vi "MatrixConfiguration.vi"() -> ()   [LabVIEW 2013]
uses:
  InstrControl/InstrumentSetup.vi
  InstrControl/InstrControl.lvclass
panel:
  in  "OK Button":bool
  in  "Apply":bool
  in  "No Matrix":bool
  in  "Save Settings":bool
  in  "Measurement":T1(ring)
  in  "Tab Control":enum32{"Pickering Matrix"}(tab)
  out "Y Mapping":string[](array[string])
  out "X Mapping":string[](array[string])
  out "Display Pickering Matrix":bool[][](array[boolean])
  out "DIAGNOSTIC? Response":string
  in  "Pickering DIAGNOSTIC?":bool
  in  "Pickering Mux2 address":i32=5 caption="Mux2 address"
  in  "Pickering Mux1 address":i32=4 caption="Mux1 address"
  in  "Pickering GPIB address":string caption="GPIB address"
  in  "Pickering Matrix address":i32=1 caption="Matrix address"
  out "X Mapping CB Standard":string[](array[string])
  # "MUX / Matrix Setup"
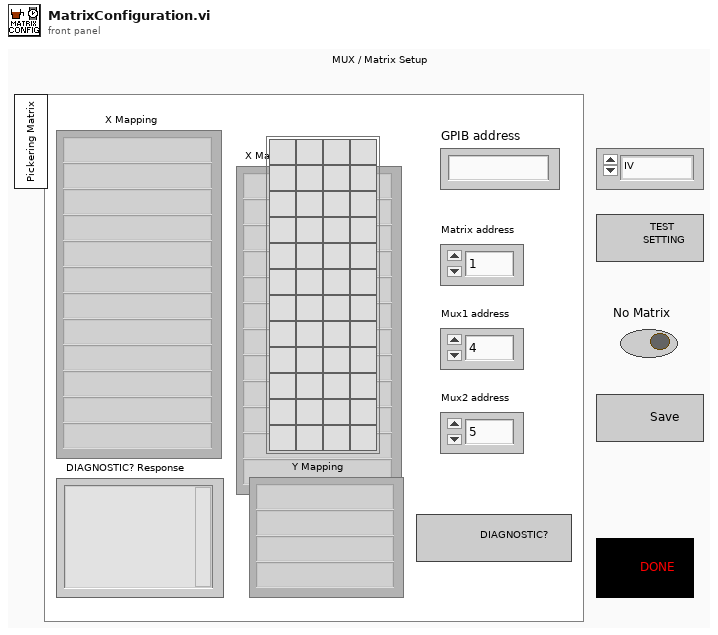
[diagram p1: front panel]
types:
  T1 = enum16{"IV", "CV", "Stability", "Striptest", "Cis", "Ris", "PTP"}
  T2 = enum16{"Reset", "Ground", "Striptest SMU", "Striptest LCR", "IV", "CV", "Interstrip Cap", "Interstrip Res"}
  T3 = cluster{"Matrix address":string, "Mux1 address":string, "Mux2 address":string, "Matrix used?":bool, "Pickering":refnum<class "Pickering.lvclass">, "Matrix X Channels":cluster{"Bias Supply / SMU LO":i32, "Bias Supply / SMU HI":i32, "CV Box LO":i32, "CV Box HI":i32, "CV Box LO IN":i32, "CV Box HI IN":i32, "Volt meter LO":i32, "Volt meter HI":i32, "Mux1 C1":i32, "Mux1 C2":i32, "Mux2 C1":i32, "Mux2 C2":i32}}
  T4 = enum16{"Left Button", "Center Button", "Right Button", "Window Close"}
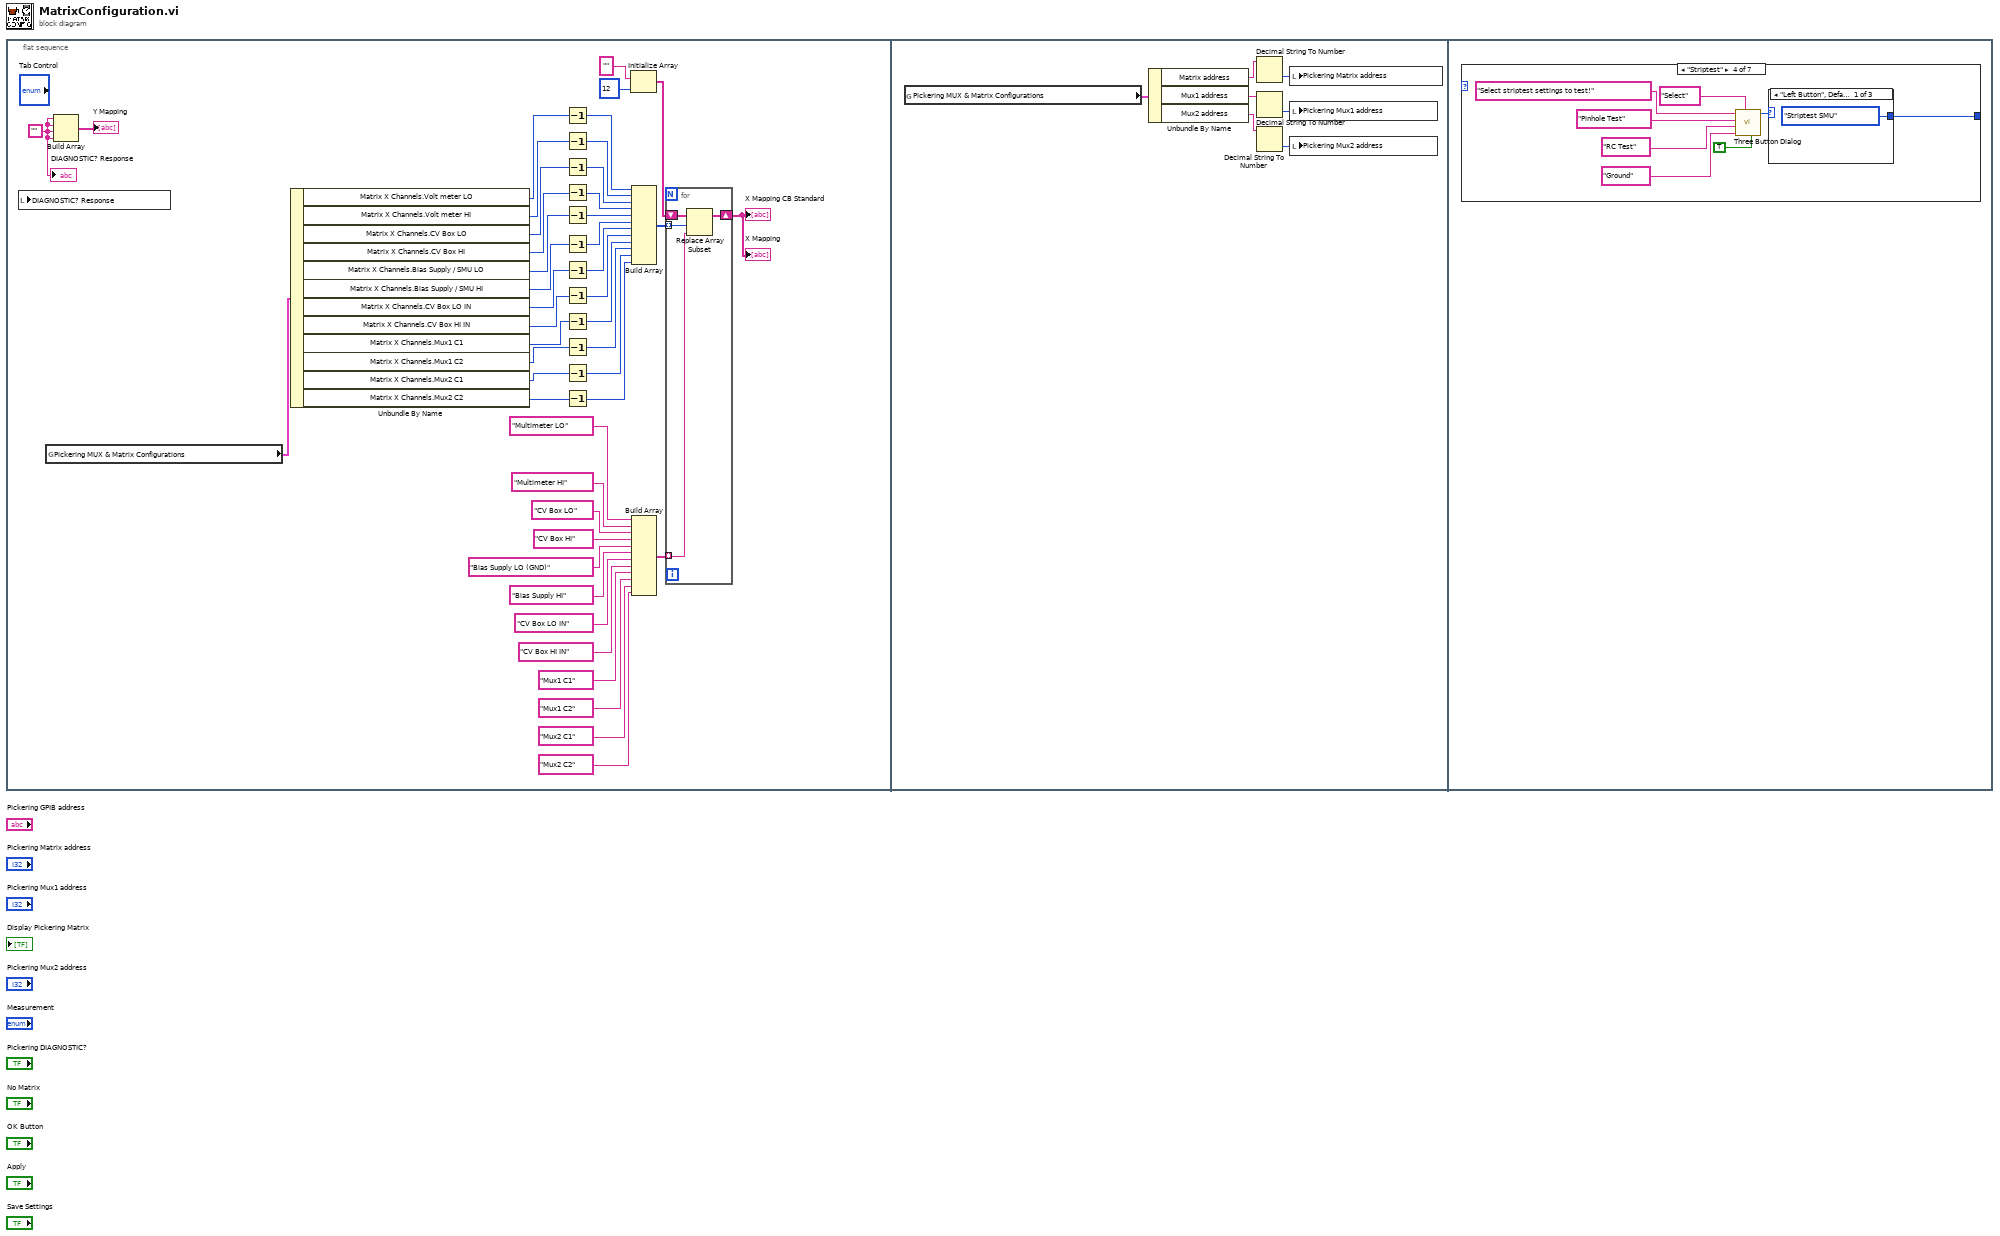
[diagram p0: block diagram]
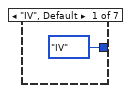
[diagram p2: hidden frame]
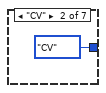
[diagram p3: hidden frame]
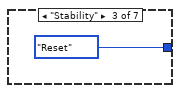
[diagram p4: hidden frame]
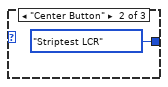
[diagram p5: hidden frame]
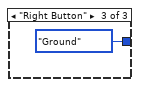
[diagram p6: hidden frame]
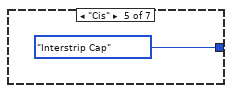
[diagram p7: hidden frame]
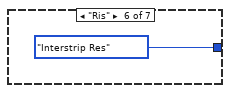
[diagram p8: hidden frame]
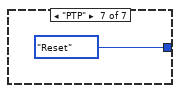
[diagram p9: hidden frame]
diagram:
  n1 = flat-sequence {
    frame #0 {
      w1 = ""
      n2 = local read "DIAGNOSTIC? Response"() -> ()  [unwired: 1 in]
      n3 = global read "InstrumentSetup.vi" "Pickering MUX & Matrix Configurations"() -> (w17:T3)
      n4 = Build Array(w1, w1, w1, w1) -> (→"Y Mapping":string[])
      n5 = Unbundle By Name(w17) -> ("Matrix X Channels.Volt meter LO"=w27:i32, "Matrix X Channels.Volt meter HI"=w29:i32, "Matrix X Channels.CV Box LO"=w18:i32, "Matrix X Channels.CV Box HI"=w23:i32, "Matrix X Channels.Bias Supply / SMU LO"=w22:i32, "Matrix X Channels.Bias Supply / SMU HI"=w21:i32, "Matrix X Channels.CV Box LO IN"=w20:i32, "Matrix X Channels.CV Box HI IN"=w19:i32, "Matrix X Channels.Mux1 C1"=w26:i32, "Matrix X Channels.Mux1 C2"=w25:i32, "Matrix X Channels.Mux2 C1"=w24:i32, "Matrix X Channels.Mux2 C2"=w4:i32)
      n6 = Decrement(x=w27) -> (x-1=w28:i32)
      n7 = Decrement(x=w29) -> (x-1=w30:i32)
      n8 = Decrement(x=w18) -> (x-1=w31:i32)
      n9 = Decrement(x=w23) -> (x-1=w32:i32)
      n10 = Decrement(x=w22) -> (x-1=w33:i32)
      n11 = Decrement(x=w21) -> (x-1=w34:i32)
      n12 = Decrement(x=w20) -> (x-1=w35:i32)
      n13 = Decrement(x=w19) -> (x-1=w36:i32)
      n14 = Decrement(x=w26) -> (x-1=w37:i32)
      n15 = Decrement(x=w25) -> (x-1=w38:i32)
      n16 = Decrement(x=w24) -> (x-1=w39:i32)
      n17 = Decrement(x=w4) -> (x-1=w40:i32)
      n18 = Initialize Array("", 12) -> (w45:string[])
      n19 = Build Array(w28, w30, w31, w32, w33, w34, w35, w36, w37, w38, w39, w40) -> (w41:i32[])
      n20 = Build Array("Multimeter LO" ("Input Element"), "Multimeter HI" ("Input Element"), "CV Box LO" ("Input Element"), "CV Box HI" ("Input Element"), "Bias Supply LO (GND)" ("Input Element"), "Bias Supply HI" ("Input Element"), "CV Box LO IN" ("Input Element"), "CV Box HI IN" ("Input Element"), "Mux1 C1" ("String"), "Mux1 C2" ("String"), "Mux2 C1" ("String"), "Mux2 C2" ("String")) -> (w42:string[])
      n21 = for {
        tunnel: w41 -> [w47] mode=indexing
        tunnel: w42 -> [w48] mode=indexing
        shift-right: [w46] -> w3
        shift-left: w45 -> [w49]
        n22 = Replace Array Subset(array=w49, new element=w48, index=w47) -> (w46:string[])
      }
      "X Mapping" <- w3
      "X Mapping CB Standard" <- w3
      "DIAGNOSTIC? Response" <- w1
    }
    frame #1 {
      n23 = global read "InstrumentSetup.vi" "Pickering MUX & Matrix Configurations"() -> (w56:T3)
      n24 = Unbundle By Name(w56) -> ("Matrix address"=w55:string, "Mux1 address"=w54:string, "Mux2 address"=w53:string)
      n25 = Decimal String To Number(string=w55) -> (number=w52:i32)  [unwired: 2 in, 1 out]
      n26 = Decimal String To Number(string=w54) -> (number=w50:i32)  [unwired: 2 in, 1 out]
      n27 = Decimal String To Number(string=w53) -> (number=w51:i32)  [unwired: 2 in, 1 out]
      n28 = local write "Pickering Matrix address"(w52) -> ()
      n29 = local write "Pickering Mux1 address"(w50) -> ()
      n30 = local write "Pickering Mux2 address"(w51) -> ()
    }
    frame #2 {
      n31 = case shown="\"Striptest\"" {
        selector: _ -> [_ _ _ _ _ _ _]
        tunnel: [T2."IV" ("Action") T2."CV" ("Action") T2."Reset" ("Action") w65 T2."Interstrip Cap" ("Action") T2."Interstrip Res" ("Action") T2."Reset" ("Action")] -> _
        frame "IV", Default {
        }
        frame "CV" {
        }
        frame "Stability" {
        }
        frame "Striptest" {
          n32 = call <vilib>:"Three Button Dialog.vi"("Allow user to close window? (TRUE)"=TRUE, "Window Title (\"\")"="Select", "Right Button Text (\"Cancel\")"="Ground", "Center Button Text (\"No\")"="RC Test", "Left Button Text (\"Yes\")"="Pinhole Test", "message"="Select striptest settings to test!") -> ("Which Button?"=w67:T4)  [unwired: 5 in]
          n33 = case shown="\"Left Button\", Default" w67 {
            tunnel: [T2."Striptest SMU" ("Action") T2."Striptest LCR" ("Action") T2."Ground" ("Action")] -> w65
            frame "Left Button", Default {
            }
            frame "Center Button" {
            }
            frame "Right Button" {
            }
          }
        }
        frame "Cis" {
        }
        frame "Ris" {
        }
        frame "PTP" {
        }
      }
    }
  }
